vi "Convert Signal to Engineering Units.vi"(8 "error in (no error)":errorcluster, 10 "Sensor CoreData":T1, 11 "Signal":dbl) -> (0 "error out":errorcluster, 3 "Measured Value":dbl)   [LabVIEW 2026, in "Processing_Engine.lvlib"]
uses:
  Processing_Engine.lvlib
  controls/UI/Units Enum.ctl
  controls/UI/Signal Enum.ctl
  controls/Messaging Payloads/Sensor CoreData Cluster.ctl
  Settings/Settings.lvlib
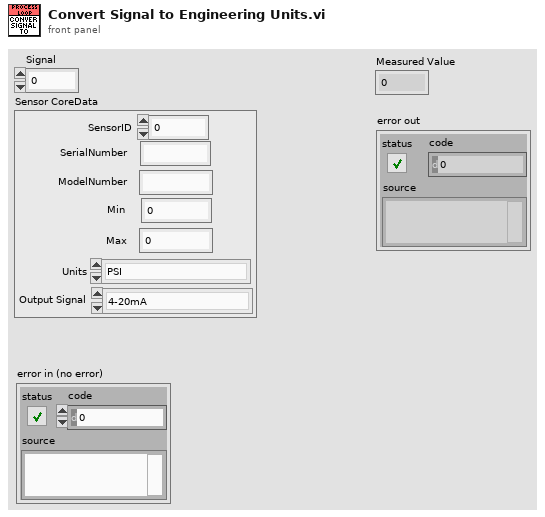
[diagram p1: front panel]
types:
  T1 = typedef "Settings.lvlib/Sensor CoreData Cluster.ctl" = cluster{"SerialNumber":string, "ModelNumber":string, "Min":dbl, "Max":dbl, "Units":T2, "Output Signal":T3, "SensorID":i32}
  T2 = typedef "Units Enum.ctl" = enum16{"PSI", "Deg C", "kPa", "GPM"}
  T3 = typedef "Signal Enum.ctl" = enum16{"4-20mA", "0-10V", "Thermocouple Type K"}
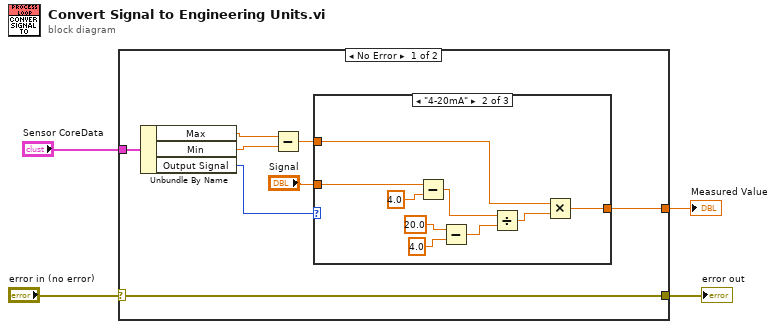
[diagram p0: block diagram]
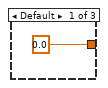
[diagram p2: hidden frame]
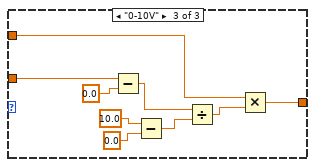
[diagram p3: hidden frame]
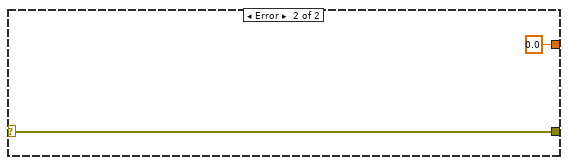
[diagram p4: hidden frame]
diagram:
  n1 = case shown="No Error" "error in (no error)" {
    selector: "error in (no error)" -> [w5 w33]
    tunnel: [w7 0.0 ("Min")] -> w4
    tunnel: "Sensor CoreData" -> [w6 _]
    tunnel: [w5 w33] -> w1
    frame No Error {
      n2 = Unbundle By Name(w6) -> ("Max"=w11:dbl, "Min"=w10:dbl, "Output Signal"=w8:T3)
      n3 = Subtract(x=w11, y=w10) -> (x-y=w9:dbl)
      n4 = case shown="\"4-20mA\"" w8 {
        tunnel: "Signal" -> [_ w17 w26]
        tunnel: w9 -> [_ w15 w24]
        tunnel: [0.0 ("Min") w14 w23] -> w7
        frame Default {
        }
        frame "4-20mA" {
          n5 = Subtract(x=w17, y=4.0) -> (x-y=w20:dbl)
          n6 = Subtract(x=20.0, y=4.0) -> (x-y=w18:dbl)
          n7 = Divide(x=w20, y=w18) -> (x/y=w16:dbl)
          n8 = Multiply(x=w15, y=w16) -> (x*y=w14:dbl)
        }
        frame "0-10V" {
          n9 = Subtract(x=w26, y=0.0) -> (x-y=w29:dbl)
          n10 = Subtract(x=10.0, y=0.0) -> (x-y=w27:dbl)
          n11 = Divide(x=w29, y=w27) -> (x/y=w25:dbl)
          n12 = Multiply(x=w24, y=w25) -> (x*y=w23:dbl)
        }
      }
    }
    frame Error {
    }
  }
  "Measured Value" <- w4
  "error out" <- w1
